vi "get Last Time222.vi"(11 "Ship in":refnum<class "Ship.lvclass">) -> (3 "Last World Update Time":dbl format="%_19f")   [LabVIEW 2015]
uses:
  Ship.lvclass
  Movable/Movable.lvclass
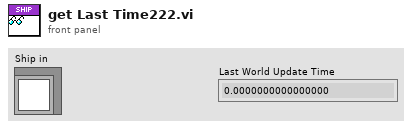
[diagram p1: front panel]
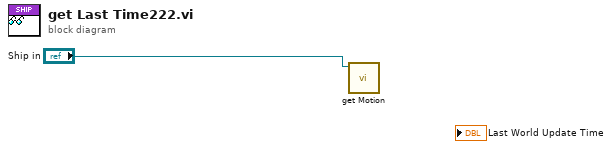
[diagram p0: block diagram]
diagram:
  n1 = call "get Motion.vi"("Movable in"="Ship in") -> ()  [unwired: 10 in, 1 out]
